vi "U3 Stream With DO.vi"() -> ()   [LabVIEW 2021]
panel:
  in  "FIO6":bool
  in  "FIO7":bool
  in  "Scan List (-)":u8[](array[numeric])=[31, 31, 31, 31, 31, 31, 31, 31, 31, 31, 31, 31, 31, 31, 31, 31, 31, 31, 31, 31, 31, 31, 31, 31, 31, 31, 31, 31, 31, 31, 31, 31, 31, 31, 31, 31, 31, 31, 31, 31, 31, 31, 31, 31, 31, 31, 31, 31, 31, 31, 31, 31, 31, 31, 31, 31, 31, 31, 31, 31, 31, 31, 31, 31, 31, 31, 31, 31, 31, 31, 31, 31, 31, 31, 31, 31, 31, 31, 31, 31, 31, 31, 31, 31, 31, 31, 31, 31, 31, 31, 31, 31, 31, 31, 31, 31, 31, 31, 31, 31, 31, 31, 31, 31, 31, 31, 31, 31, 31, 31, 31, 31, 31, 31, 31, 31, 31, 31, 31, 31, 31, 31, 31, 31, 31, 31, 31, 31]
  out "Waveform Graph":dbl[][](graph)
  in  "Scan List (+)":u8[](array[numeric])=[0, 1, 2, 3]
  out "Actual Scan Rate (Hz)":dbl=1000.0 format="%.3f"
  out "# Scans Read":i32
  out "# of iterations":i32
  out "Data":dbl[][](array[numeric]) format="%.3f"
  in  "Scan Rate (Hz)":dbl=1000.0 format="%.3f"
  in  "stop":bool
  out "Error Message":string
  # "This example streams from the first found USB U3.  Streaming\nrequires U3 hardware revision 1.21+."
  # "The + scan list is the positive\nchannels.  For each element in\nthe + list, there must also be\nan element in the - list, which is\nthe negative channels.  For\nsingle-ended channels, put in\n31 for the negative channel."
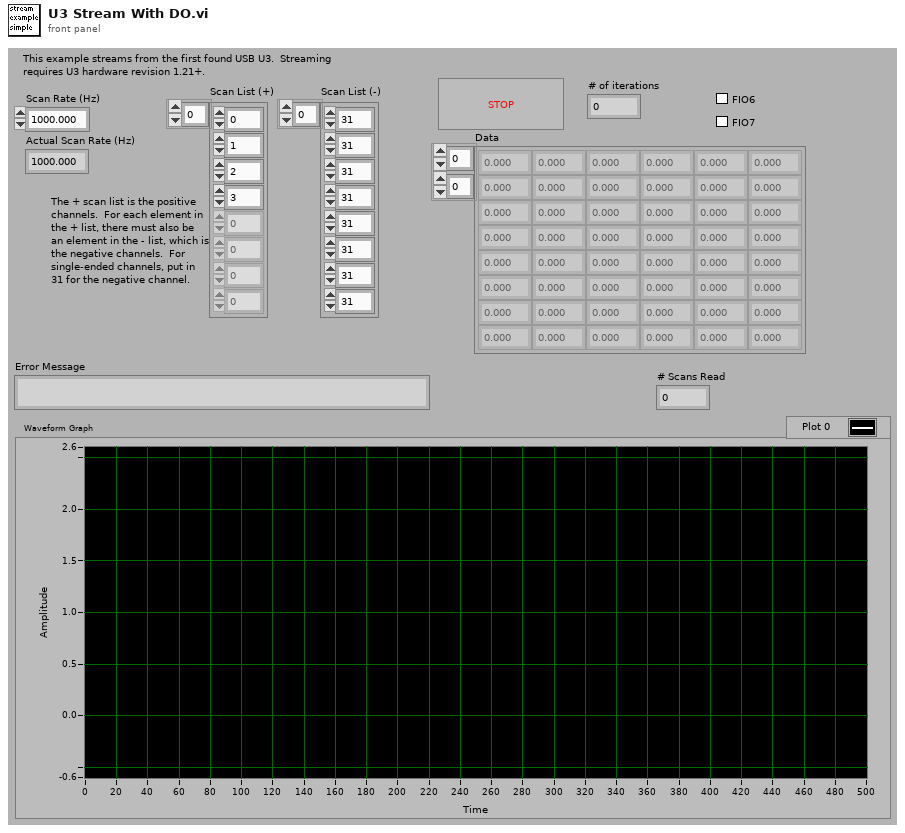
[diagram p1: front panel]
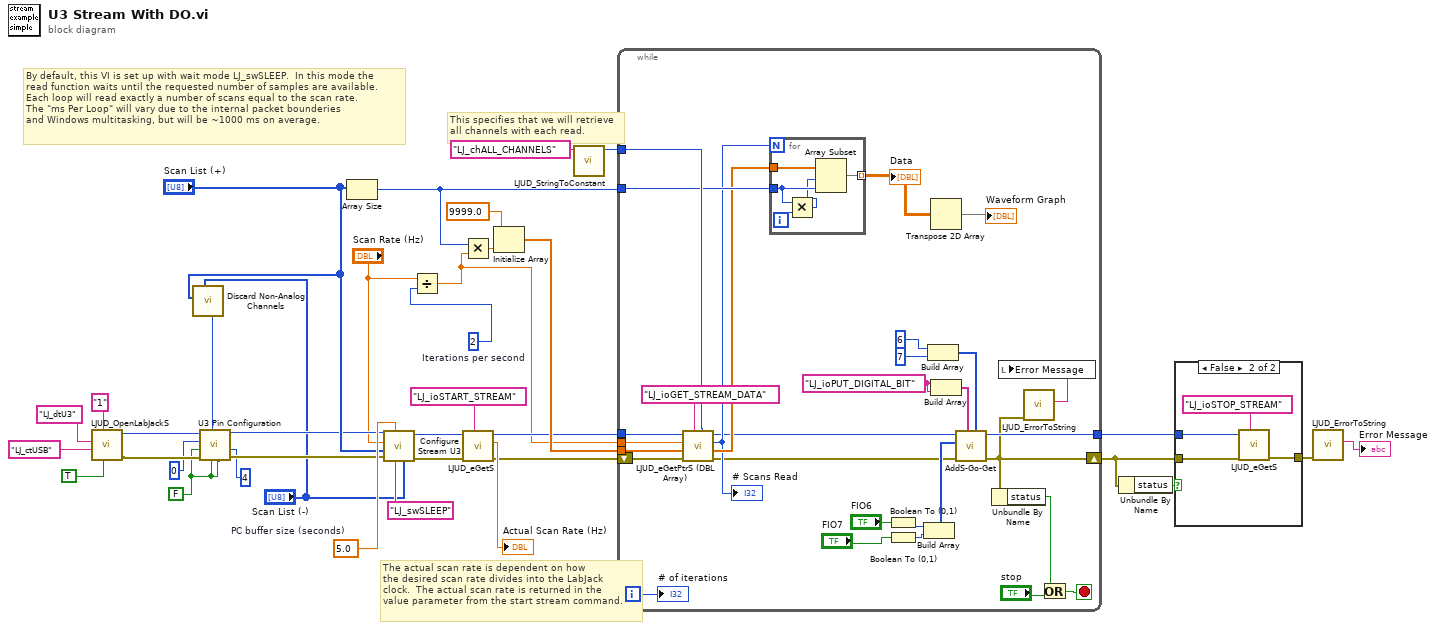
[diagram p0: block diagram]
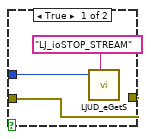
[diagram p2: hidden frame]
diagram:
  w3 = 2  # Iterations per second
  w14 = FALSE ("Enable DAC1")
  w26 = 5.0  # PC buffer size (seconds)
  # "This specifies that we will retrieve\nall channels with each read."
  # "The actual scan rate is dependent on how\nthe desired scan rate divides into the LabJack\nclock.  The actual scan rate is returned in the\nvalue parameter from the start stream command."
  # "By default, this VI is set up with wait mode LJ_swSLEEP.  In this mode the\nread function waits until the requested number of samples are available.\nEach loop will read exactly a number of scans equal to the scan rate.\nThe \"ms Per Loop\" will vary due to the internal packet bounderies\nand Windows multitasking, but will be ~1000 ms on average."
  n1 = call "LJUD_OpenLabJackS.vi"("FirstFound"=TRUE, "Address"="1", "ConnectionType"="LJ_ctUSB", "DeviceType"="LJ_dtU3") -> ("error out"=w17:errorcluster, "Handle"=w18:i32)  [unwired: 5 in, 1 out]
  n2 = call "Discard Non-Analog Channels.vi"("Channels In (-)"="Scan List (-)", "Channels In"="Scan List (+)") -> ("FIO/EIO Analog Enable"=w13:i32)  [unwired: 6 in, 3 out]
  n3 = call "U3 Pin Configuration.vi"("Timer/Counter Pin Offset"=u8 4, "Enable Counter1"=w14, "Enable Counter0"=w14, "FIO/EIO Analog Enable"=w13, "error in"=w17, "Enable DAC1"=w14, "Number of Timers Enabled"=u8 0, "Handle In"=w18) -> ("error out"=w10:errorcluster, "Handle Out"=w11:i32)  [unwired: 2 in]
  n4 = Array Size(array="Scan List (+)") -> (size(s)=w30:i32)
  n5 = call "Configure Stream U3.vi"("Scan List (-)"="Scan List (-)", "Wait Mode"="LJ_swSLEEP" ("Wait Mode (2)"), "PC buffer size (seconds)"=w26, "error in"=w10, "Scan List (+)"="Scan List (+)", "Scan Rate (Hz)"="Scan Rate (Hz)", "Handle In"=w11) -> ("error out"=w34:errorcluster, "Handle Out"=w35:i32)  [unwired: 2 in, 1 out]
  n6 = Divide(x="Scan Rate (Hz)", y=w3) -> (x/y=w2:dbl)
  n7 = Multiply(x=w30, y=w2) -> (x*y=w33:dbl)
  n8 = call "LJUD_eGetS.vi"("IOType"="LJ_ioSTART_STREAM", "error in"=w34, "Handle In"=w35) -> ("error out"=w20:errorcluster, "Value Read"=→"Actual Scan Rate (Hz)":dbl, "Handle Out"=w24:i32)  [unwired: 6 in]
  n9 = Initialize Array(9999.0, w33) -> (w31:dbl[])
  n10 = call "LJUD_StringToConstant.vi"("String"="LJ_chALL_CHANNELS") -> ("Constant Number"=w21:i32)  [unwired: 9 in, 1 out]
  n11 = while {
    tunnel: [w39] -> w7
    shift-left: w20 -> [w57]
    shift-right: [w38] -> w19
    tunnel: w21 -> [w58]
    tunnel: w30 -> [w54]
    tunnel: w31 -> [w61]
    tunnel: w2 -> [w60]
    tunnel: w24 -> [w63]
    i -> [w59]
    stop <- w64 stop-if-true
    w51 = "LJ_ioPUT_DIGITAL_BIT" ("IOType")
    n12 = call "LJUD_eGetPtrS (DBL Array).vi"("Channel"=w58, "IOType"="LJ_ioGET_STREAM_DATA", "error in"=w57, "DBL Array Write"=w61, "Value"=w60, "Handle In"=w63) -> ("error out"=w41:errorcluster, "DBL Array Read"=w53:dbl[], "Value"=w52:i32, "Handle Out"=w40:i32)  [unwired: 2 in]
    "# Scans Read" <- w52
    n13 = for {
      N: w52 -> [_]
      tunnel: w53 -> [w71]
      tunnel: w54 -> [w70]
      tunnel: [w67] -> w55 mode=indexing
      i -> [w69]
      n14 = Multiply(x=w70, y=w69) -> (x*y=w68:i32)
      n15 = Array Subset(array=w71, index=w68, length=w70) -> (w67:dbl[])
    }
    "Data" <- w55
    n16 = Boolean To (0,1)(Boolean="FIO6") -> (0, 1=w46:i16)
    n17 = Boolean To (0,1)(Boolean="FIO7") -> (0, 1=w45:i16)
    n18 = Build Array(w46, w45) -> (w44:i16[])
    n19 = Build Array(6, 7) -> (w49:i32[])
    n20 = Transpose 2D Array(2D array=w55) -> (transposed array=→"Waveform Graph":dbl[][])
    n21 = Build Array(w51, w51) -> (w50:string[])
    n22 = call "AddS-Go-Get.vi"("Channels"=w49, "IOTypes"=w50, "error in"=w41, "Values Write"=w44, "Handle In"=w40) -> ("error out"=w38:errorcluster, "Handle Out"=w39:i32)  [unwired: 4 in, 1 out]
    n23 = Unbundle By Name(w38) -> ("status"=w65:bool)
    n24 = call "LJUD_ErrorToString.vi"("error in"=w38) -> ("String"=w37:string)  [unwired: 10 in]
    n25 = local write "Error Message"(w37) -> ()
    n26 = Or(x=w65, y="stop") -> (x .or. y?=w64:bool)
    "# of iterations" <- w59
  }
  n27 = Unbundle By Name(w19) -> ("status"=w23:bool)
  n28 = case shown="False" w23 {
    tunnel: [w73 w77] -> w28
    tunnel: w19 -> [w73 w76]
    tunnel: w7 -> [w72 w75]
    frame True {
      n29 = call "LJUD_eGetS.vi"("IOType"="LJ_ioSTOP_STREAM", "Handle In"=w72) -> ()  [unwired: 7 in, 3 out]
    }
    frame False {
      n30 = call "LJUD_eGetS.vi"("IOType"="LJ_ioSTOP_STREAM", "error in"=w76, "Handle In"=w75) -> ("error out"=w77:errorcluster)  [unwired: 6 in, 2 out]
    }
  }
  n31 = call "LJUD_ErrorToString.vi"("error in"=w28) -> ("String"=→"Error Message":string)  [unwired: 10 in]
